vi "Get Scene Item ID.vi"(7 "Search Offset (0)":i32, 8 "error in (no error)":errorcluster, 9 "Source Name":string, 10 "Scene Name":string, 11 "OBS in":refnum<class "OBS.lvclass">) -> (0 "error out":errorcluster, 2 "Scene Item ID":i32, 3 "OBS out":refnum<class "OBS.lvclass">)   [LabVIEW 2022 SP3, in "obs-websocket-lv.lvlib" / "OBS.lvclass"]
uses:
  OBS.lvclass
  OBS.lvclass/OBS.ctl
  GetSceneItemID/GetSceneItemID.lvclass
  RGetSceneItemID/RGetSceneItemID.lvclass
  C:/dev/illuminatedg/obs-websocket-lv/obs-websocket-lv/Response/Response.lvclass
  C:/dev/illuminatedg/obs-websocket-lv/obs-websocket-lv/Server Message/Server Message.lvclass
  C:/dev/illuminatedg/obs-websocket-lv/obs-websocket-lv/Message/Message.lvclass
  C:/dev/illuminatedg/obs-websocket-lv/obs-websocket-lv/RGetSceneItemID/RGetSceneItemID.lvclass
  C:/dev/illuminatedg/obs-websocket-lv/obs-websocket-lv/Request/Request.lvclass
  C:/dev/illuminatedg/obs-websocket-lv/obs-websocket-lv/Client Message/Client Message.lvclass
  C:/dev/illuminatedg/obs-websocket-lv/obs-websocket-lv/GetSceneItemID/GetSceneItemID.lvclass
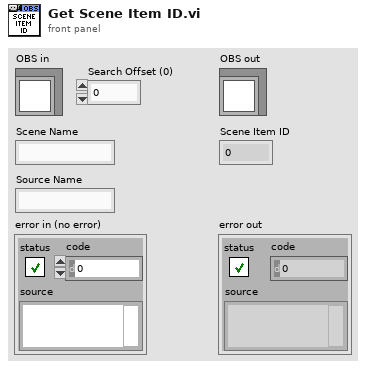
[diagram p1: front panel]
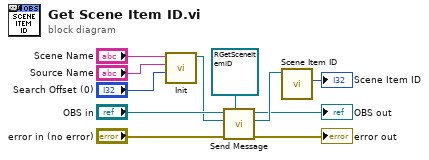
[diagram p0: block diagram]
diagram:
  n1 = call "Init.vi"("Search Offset (0)"="Search Offset (0)", "Source Name"="Source Name", "Scene Name"="Scene Name") -> ("GetSceneItemID out"=w6:refnum<class "GetSceneItemID.lvclass">)  [unwired: 7 in, 1 out]
  n2 = call "Send Message.vi"("Response Type (None)"=refnum<class "RGetSceneItemID.lvclass"> refnum ("obs-websocket-lv.lvlib:RGetSceneItemID.lvclass"), "error in (no error)"="error in (no error)", "Client Message"=w6, "OBS in"="OBS in") -> ("error out"=→"error out":errorcluster, "Response"=w4:refnum<class "RGetSceneItemID.lvclass">, "OBS out"=→"OBS out":refnum<class "OBS.lvclass">)  [unwired: 4 in, 1 out]
  n3 = call "Scene Item ID.vi"("RGetSceneItemID in"=w4) -> ("Scene Item ID"=→"Scene Item ID":i32)  [unwired: 8 in, 2 out]
